vi "Post No-Rep Message.vi"(6 "Response Timeout(5000ms)":i32=5000, 7 "TcpRouter-Client in":refnum<class "TcpRouter-Client.lvclass">, 8 "error in (no error)":errorcluster, 9 "Target Module":string="Target", 10 "Arguments (\"\")":string, 11 "State":string="API State") -> (0 "error out":errorcluster)   [LabVIEW 2020, in "CSM-TCP-Router.lvlib" / "TcpRouter-Client.lvclass"]
uses:
  TcpRouter-Client.lvclass
  _support/tcp-msg type.ctl
  <userlib>/_NEVSTOP/Communicable State Machine(CSM)/_Polymophic/Build No-Reply Asynchronous Message with Arguments.vi
  f32241c3-0036-4787-bc41-e9c1f987f5e1.vi
  <userlib>/_NEVSTOP/Communicable State Machine(CSM)/AdvanceAPI/CSM - Revert Arguments-Safe String.vi
  <userlib>/_NEVSTOP/Communicable State Machine(CSM)/AdvanceAPI/CSM - Keywords.vi
  <userlib>/_NEVSTOP/Communicable State Machine(CSM)/_Support/Message/Parse State with Arguments String.vi
  <userlib>/_NEVSTOP/Communicable State Machine(CSM)/_Shared/Trim Single-line Text.vi
  CSM-TCP-Router.lvlib
  <userlib>/_NEVSTOP/Communicable State Machine(CSM)/Communicable State Machine.lvlib
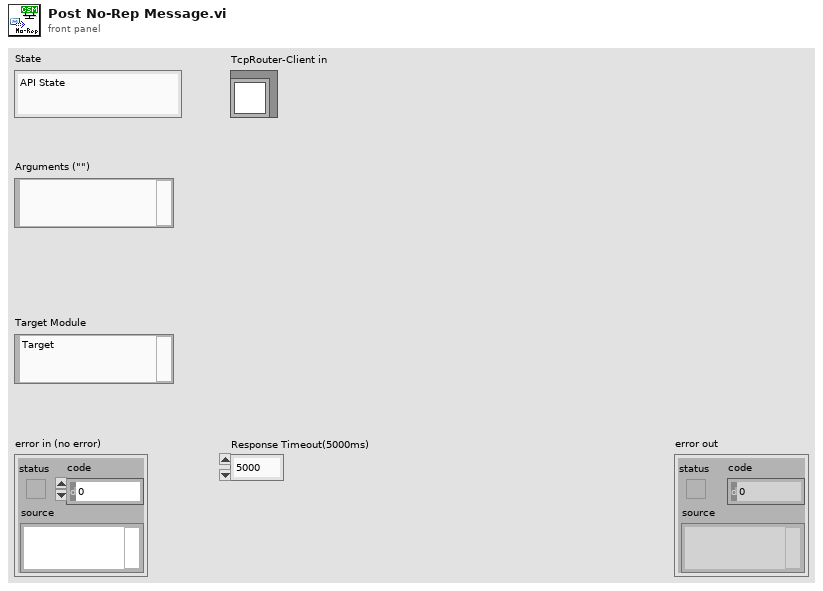
[diagram p1: front panel]
types:
  T1 = typedef "CSM-TCP-Router.lvlib/tcp-msg type.ctl" = enum8{"info", "error", "cmd", "cmd-resp", "resp", "async-resp", "status", "interrupt"}
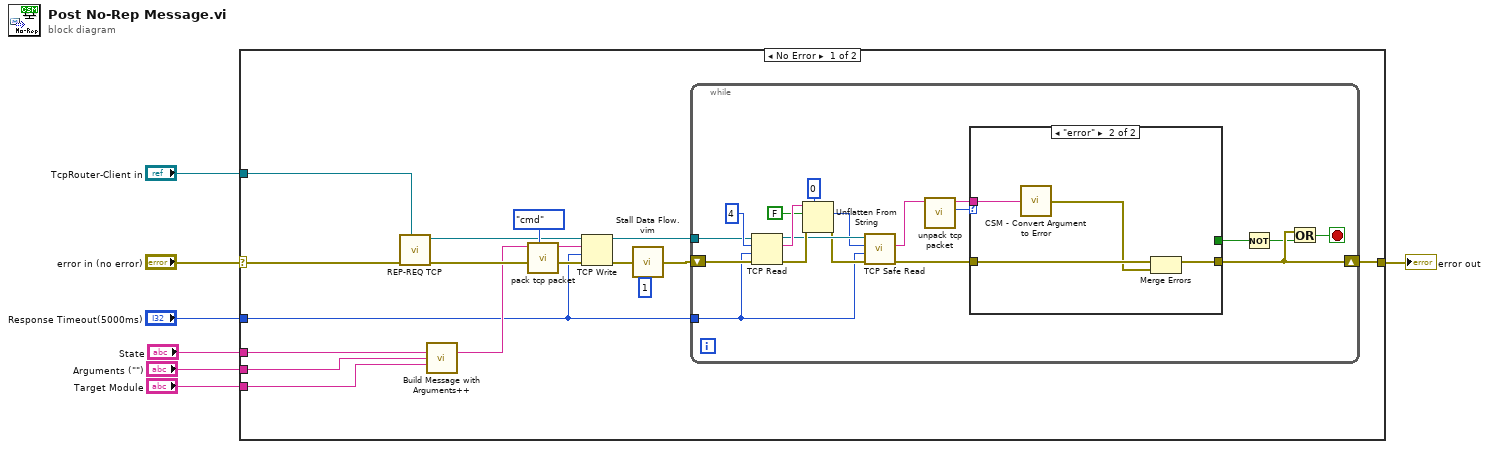
[diagram p0: block diagram]
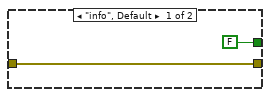
[diagram p2: hidden frame]
diagram:
  n1 = case shown="No Error" "error in (no error)" {
    selector: "error in (no error)" -> [w23 w49]
    tunnel: [w9 w49] -> w6
    tunnel: "TcpRouter-Client in" -> [w22 _]
    tunnel: "Response Timeout(5000ms)" -> [w8 _]
    tunnel: "State" -> [w17 _]
    tunnel: "Arguments (\"\")" -> [w16 _]
    tunnel: "Target Module" -> [w15 _]
    frame No Error {
      n2 = call "REP-REQ TCP.vi"("TcpRouter-Client in"=w22, "error in (no error)"=w23) -> ("error out"=w19:errorcluster, "connection ID"=w18:refnum<k5>)  [unwired: 7 in, 1 out]
      n3 = call-poly <userlib>:"Build Message with Arguments++.vi"("State with Arguments"=w17, "Arguments (\"\")"=w16, "Target Module (\"\")"=w15) -> ("CSM Message String"=w14:string)  [unwired: 12 in]
      n4 = call "pack tcp packet.vi"("tcp-message-type"=tcp-msg_type."cmd", "String"=w14) -> ("TCP Pack"=w21:string)  [unwired: 9 in]
      n5 = TCP Write(connection ID=w18, data in=w21, error in (no error)=w19, 9:w8) -> (connection ID out=w11:refnum<k5>, error out=w13:errorcluster)  [unwired: 1 out]
      n6 = call "Stall Data Flow.vim"("value in"=w13, "milliseconds to wait"=u32 1) -> ("value out"=w10:errorcluster)  [unwired: 1 out]
      n7 = while {
        tunnel: w11 -> [w33]
        shift-right: [w28] -> w9
        shift-left: w10 -> [w32]
        tunnel: w8 -> [w27]
        stop <- w26 stop-if-true
        n8 = TCP Read(connection ID=w33, bytes to read=4, error in (no error)=w32, 9:w27) -> (connection ID out=w40:refnum<k5>, data out=w41:string, error out=w42:errorcluster)  [unwired: 1 in]
        n9 = Unflatten From String(type=0, binary string=w41, data includes array or string size? (T)=FALSE, error in (no error)=w42) -> (value=w38:i32, error out=w37:errorcluster)  [unwired: 2 out]
        n10 = call "TCP Safe Read.vi"("error in (no error)"=w37, "timeout ms (25000)"=w27, "bytes to read"=w38, "TCP Network Connection in"=w40) -> ("error out"=w30:errorcluster, "String"=w39:string)  [unwired: 5 in, 1 out]
        n11 = call "unpack tcp packet.vi"("TCP Pack"=w39) -> ("tcp-message-type"=w31:T1, "String"=w29:string)  [unwired: 9 in]
        n12 = case shown="\"error\"" w31 {
          tunnel: w30 -> [w44 w48]
          tunnel: [w44 w46] -> w28
          tunnel: w29 -> [_ w47]
          tunnel: [FALSE _] -> w25
          frame "info", Default {
          }
          frame "error" {
            n13 = call <userlib>:"CSM - Convert Argument to Error.vi"("Argument"=w47) -> ("error"=w45:errorcluster)  [unwired: 4 in]
            n14 = Merge Errors(w48, w45) -> (w46:errorcluster)
          }
        }
        n15 = Not(x=w25) -> (.not. x?=w24:bool)
        n16 = Or(x=w28, y=w24) -> (x .or. y?=w26:bool)
      }
    }
    frame Error {
    }
  }
  "error out" <- w6
